vi "BORRADO_MEJORADO_Gonzalo.vi"(9 "Bytes LIBRE OK":i64, 11 "Bytes Minimo de Memoria libre":i64) -> ()   [LabVIEW 2015]
panel:
  out "last mod":timestamp
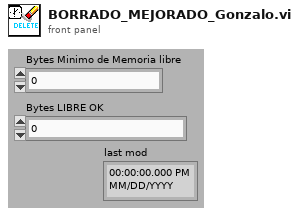
[diagram p1: front panel]
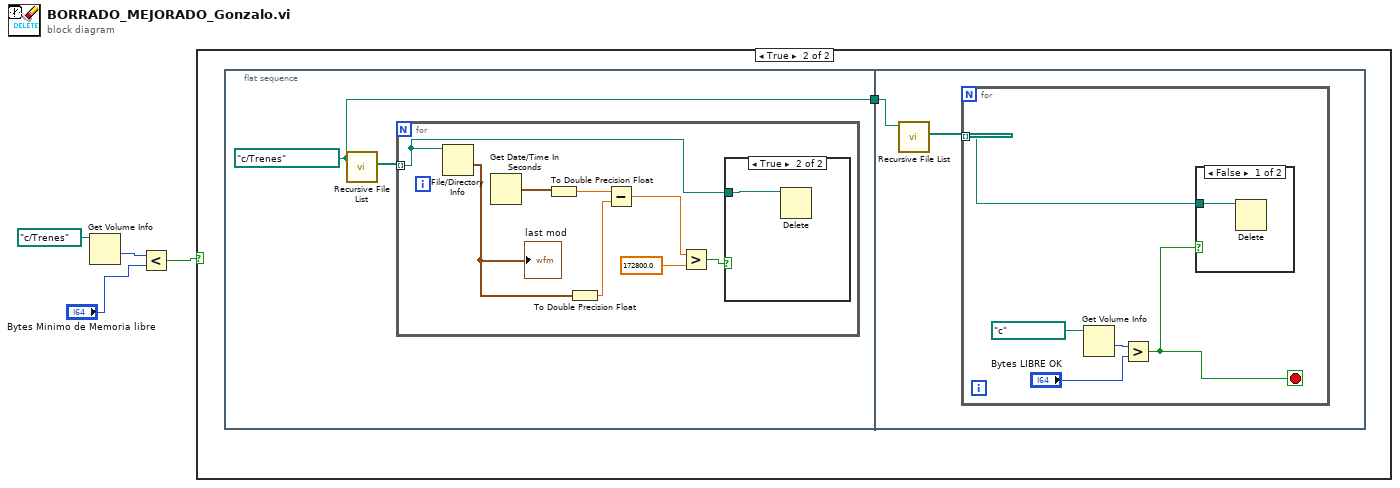
[diagram p0: block diagram]
diagram:
  n1 = Get Volume Info(11:path "c:/Trenes" ("path")) -> (1:w3:i64)  [unwired: 1 in, 5 out]
  n2 = Less?(x=w3, y="Bytes Minimo de Memoria libre") -> (x < y?=w1:bool)
  n3 = case shown="True" w1 {
    frame False {
    }
    frame True {
      n4 = flat-sequence {
        tunnel: [w6] -> w5
        tunnel: w5 -> [w18]
        frame #0 {
          w6 = path "c:/Trenes" ("path")
          n5 = call <vilib>:"Recursive File List.vi"("Folder Path"=w6) -> ("All Files in Dir"=w7:path[])  [unwired: 6 in, 4 out]
          n6 = for {
            tunnel: w7 -> [w9] mode=indexing
            n7 = File/Directory Info(path=w9) -> (last mod=w11:timestamp)  [unwired: 1 in, 6 out]
            "last mod" <- w11
            n8 = Get Date/Time In Seconds() -> (seconds since 1Jan1904=w13:timestamp)
            n9 = To Double Precision Float(number=w13) -> (double precision float=w15:dbl)
            n10 = To Double Precision Float(number=w11) -> (double precision float=w14:dbl)
            n11 = Subtract(x=w15, y=w14) -> (x-y=w8:dbl)
            n12 = Greater?(x=w8, y=172800.0) -> (0:w10:bool)
            n13 = case shown="True" w10 {
              tunnel: w9 -> [_ w16]
              frame False {
              }
              frame True {
                n14 = Delete(path (use dialog)=w16) -> ()  [unwired: 4 in, 3 out]
              }
            }
          }
        }
        frame #1 {
          n15 = call <vilib>:"Recursive File List.vi"("Folder Path"=w18) -> ("All Files in Dir"=w17:path[])  [unwired: 6 in, 4 out]
          n16 = for {
            tunnel: w17 -> [w21] mode=indexing
            stop <- w19 stop-if-true
            n17 = Get Volume Info(11:path "c:/" ("path")) -> (1:w23:i64)  [unwired: 1 in, 5 out]
            n18 = Greater?(x=w23, y="Bytes LIBRE OK") -> (0:w19:bool)
            n19 = case shown="False" w19 {
              tunnel: w21 -> [w24 _]
              frame False {
                n20 = Delete(path (use dialog)=w24) -> ()  [unwired: 4 in, 3 out]
              }
              frame True {
              }
            }
          }
        }
      }
    }
  }
